vi "Write Skip Fire Setup.vi"(8 "error in (no error)":errorcluster, 10 "Skip Fire Setup":T1[](array[typedef]), 11 "DCM-DSI-HW in":refnum<class "DCM-DSI.lvclass">) -> (0 "error out":errorcluster, 3 "DCM-DSI-HW out":refnum<class "DCM-DSI.lvclass">)   [LabVIEW 2016, in "DCM-DSI.lvclass"]
uses:
  DCM-DSI.lvclass
  <vilib>/Powertrain Controls/Device Drivers/DCM/Skip Fire/RT/Skip Fire Setup.ctl
  DCM-DSI.lvclass/DCM-DSI.ctl
  <vilib>/Powertrain Controls/Device Drivers/DCM/Skip Fire/RT/DCM - RT - Skip Fire.lvlib
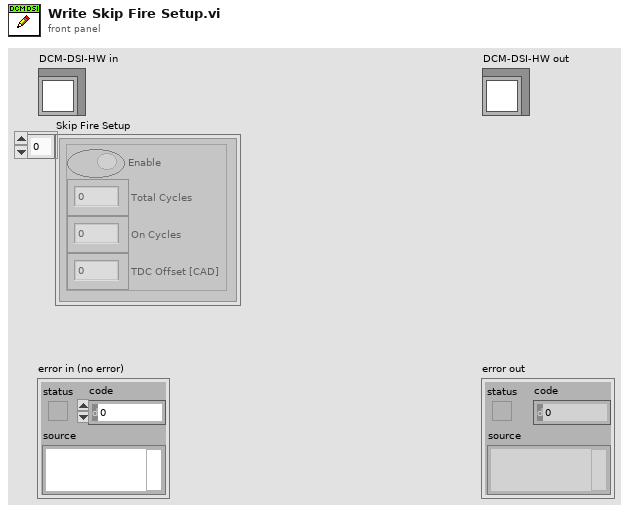
[diagram p1: front panel]
types:
  T1 = typedef "DCM - RT - Skip Fire.lvlib/Skip Fire Setup.ctl" = cluster{"Enable":bool, "Total Cycles":u8, "On Cycles":u8, "TDC Offset [CAD]":sgl}
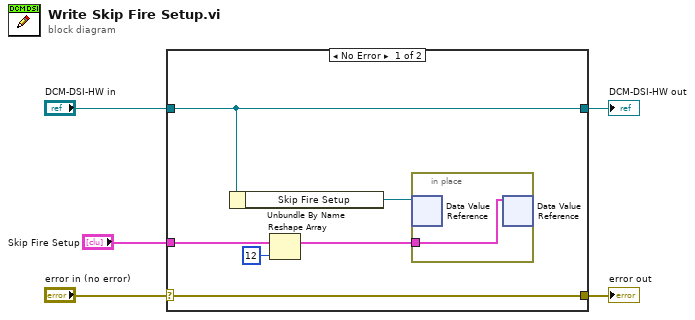
[diagram p0: block diagram]
diagram:
  n1 = case shown="No Error" "error in (no error)" {
    selector: "error in (no error)" -> [w11 w14]
    tunnel: [w11 w14] -> w4
    tunnel: [w9 w13] -> w2
    tunnel: "DCM-DSI-HW in" -> [w9 w13]
    tunnel: "Skip Fire Setup" -> [w8 _]
    frame No Error {
      n2 = Unbundle By Name(w9) -> ("Skip Fire Setup"=w10:refnum<data-value>)
      n3 = Reshape Array(w8, 12 ("dimension size")) -> (w7:T1[])
      n4 = in-place {
        in-place-border: w7 -> [w12]
        n5 = in-place-dvr #1(w10) -> ()  [unwired: 2 out]
        n6 = in-place-dvr #1(w12) -> ()  [unwired: 2 out]
      }
    }
    frame Error {
    }
  }
  "error out" <- w4
  "DCM-DSI-HW out" <- w2
